vi "Call Function.vi"(7 "Function Name":string, 8 "error in (no error)":errorcluster, 9 "Arguments (Default -Empty)":T1[](array[typedef]), 11 "Data Value Reference in":refnum<data-value>) -> (0 "error out":errorcluster, 2 "Returned Python Object Refnum":T1, 3 "Data Value Reference out":refnum<data-value>)   [LabVIEW 2020, in "G-Embedded-Python-Interpreter-Toolkit.lvlib"]
uses:
  G-Embedded-Python-Interpreter-Toolkit.lvlib
  Python Object Reference.ctl
  Python Object Type.ctl
  Merge Call Library Errors.vi
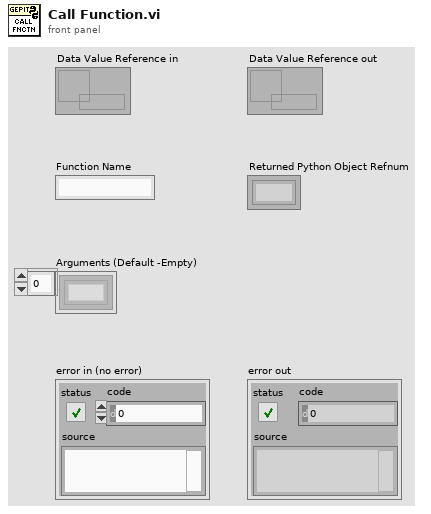
[diagram p1: front panel]
types:
  T1 = typedef "G-Embedded-Python-Interpreter-Toolkit.lvlib/Python Object Reference.ctl" = refnum<k1>
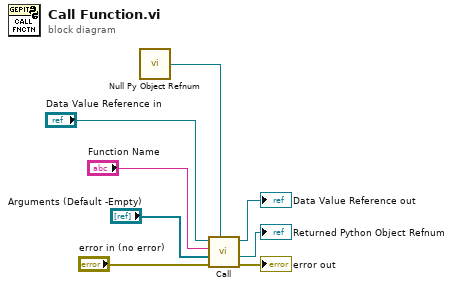
[diagram p0: block diagram]
diagram:
  n1 = call "Null Py Object Refnum.vi"() -> ("Null Python Object Refnum"=w1:T1)
  n2 = call "Call.vi"("Class Instance"=w1, "error in (no error)"="error in (no error)", "Arguments"="Arguments (Default -Empty)", "Function/Method Name"="Function Name", "Session Handle in"="Data Value Reference in") -> ("error out"=→"error out":errorcluster, "Returned Python Object Refnum"=→"Returned Python Object Refnum":T1, "Session Handle out"=→"Data Value Reference out":refnum<data-value>)  [unwired: 4 in]
